vi "Parent Class Setup.vi"(8 "error in (no error)":errorcluster, 10 "String":string) -> (0 "error out":errorcluster, 3 "class string out":refnum<class "Parent.lvclass">)   [LabVIEW 2023]
doc: "This VI accesses to Parent.ctl, the data member of Parent.lvclass, by calling the Write String Data VI.\n\nUse this VI as a setup VI for the Add Prefix.lvtest test."
uses:
  Parent.lvclass
panel:
  # "Overview:\nThis VI accesses to Parent.ctl, the data member of Parent.lvclass, by calling the Write String Data VI.\nUse this VI as a setup VI for the Add Prefix.lvtest test."
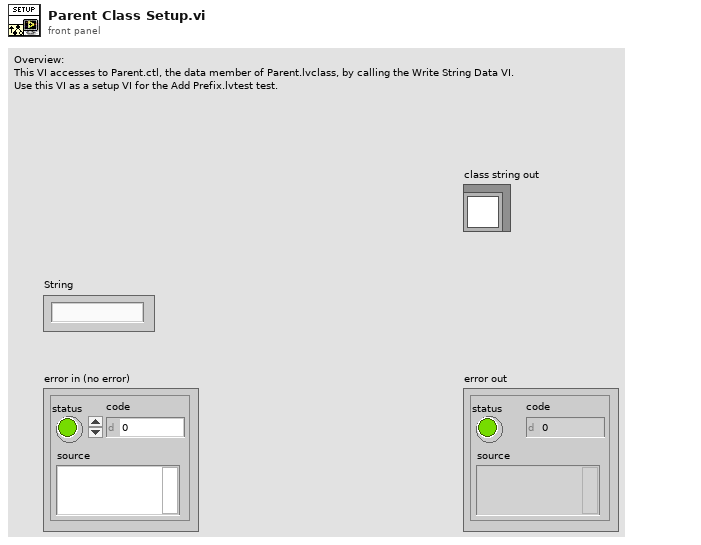
[diagram p1: front panel]
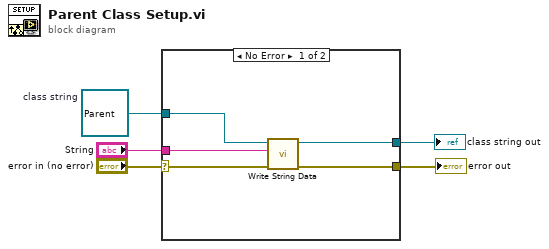
[diagram p0: block diagram]
diagram:
  w1 = refnum<class "Parent.lvclass"> refnum  # class string
  n1 = case shown="No Error" "error in (no error)" {
    selector: "error in (no error)" -> [w7 w12]
    tunnel: "String" -> [w10 _]
    tunnel: [w9 w11] -> w4
    tunnel: [w8 w12] -> w3
    tunnel: w1 -> [w6 w11]
    frame No Error {
      n2 = call-dynamic "Write String Data.vi"("error in (no error)"=w7, "String Data"=w10, "class string in"=w6) -> ("error out"=w8:errorcluster, "class string out"=w9:refnum<class "Parent.lvclass">)  [unwired: 7 in]
    }
    frame Error {
    }
  }
  "class string out" <- w4
  "error out" <- w3
